vi "Create Linear Vector by Samples.vi"(8 "error in (no error)":errorcluster, 9 "Samples":i32=128, 10 "Stop":dbl=1.0, 11 "Start":dbl) -> (0 "error out":errorcluster, 2 "Count":i32, 3 "Vector":dbl[](array[numeric]))   [LabVIEW 2017]
uses:
  <vilib>/Analysis/1siggen.llb/Ramp Pattern by Samples.vi
  <vilib>/Analysis/NI_AALBase.lvlib
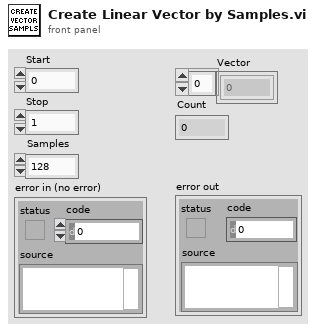
[diagram p1: front panel]
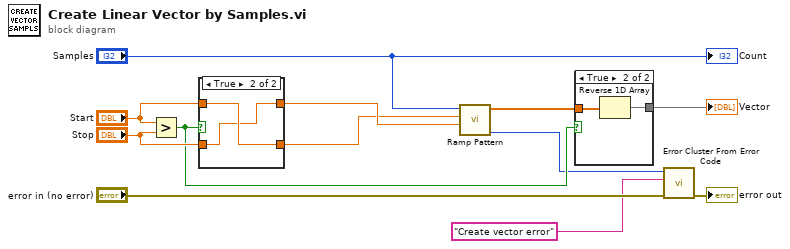
[diagram p0: block diagram]
diagram:
  n1 = Greater?(x="Start", y="Stop") -> (0:w7:bool)
  n2 = case shown="True" w7 {
    tunnel: "Start" -> [w14 w16]
    tunnel: "Stop" -> [w13 w15]
    tunnel: [w14 w15] -> w10
    tunnel: [w13 w16] -> w9
    frame False {
    }
    frame True {
    }
  }
  n3 = call-poly <vilib>:"Ramp Pattern.vi"("start"=w10, "end"=w9, "samples"="Samples") -> ("error"=w5:i32, "Ramp Pattern"=w8:dbl[])  [unwired: 7 in]
  n4 = case shown="True" w7 {
    tunnel: w8 -> [w17 w19]
    tunnel: [w17 w18] -> w6
    frame False {
    }
    frame True {
      n5 = Reverse 1D Array(array=w19) -> (reversed array=w18:dbl[])
    }
  }
  "Vector" <- w6
  n6 = call <vilib>:"Error Cluster From Error Code.vi"("error in (no error)"="error in (no error)", "error message (\"\")"="Create vector error" ("error message (\"\")"), "error code (0)"=w5) -> ("error out"=→"error out":errorcluster)  [unwired: 6 in]
  "Count" <- "Samples"
